vi "Kinimatics_Matrix_CoerceSize.vi"(9 "Columns":i32, 10 "Rows":i32, 11 "input matrix":T1) -> (0 "Coerced":bool, 3 "output matrix":T1)   [LabVIEW 2020, in "Swerve_Odometry_SEN.lvlib"]
doc: "Ensure a matrix is the size that is needed.\n\nInputs:\n - Input Matrix -- The matrix to be checked and resized if needed\n - Rows -- The expected number of rows\n - Columns -- The expected number of columns\n\nOutputs:\n - Output Matrix -- The potentially resized matrix\n - Coerced -- If TRUE, the matrix size was modified."
uses:
  <vilib>/Analysis/Matrix/Datatypes/RealMatrix.ctl
  Swerve_Odometry_SEN.lvlib
  <vilib>/Analysis/Matrix/NI_Matrix.lvlib
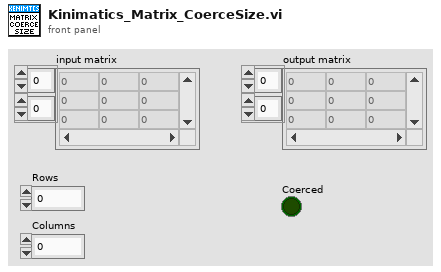
[diagram p1: front panel]
types:
  T1 = typedef "NI_Matrix.lvlib/RealMatrix.ctl" = dbl[][]
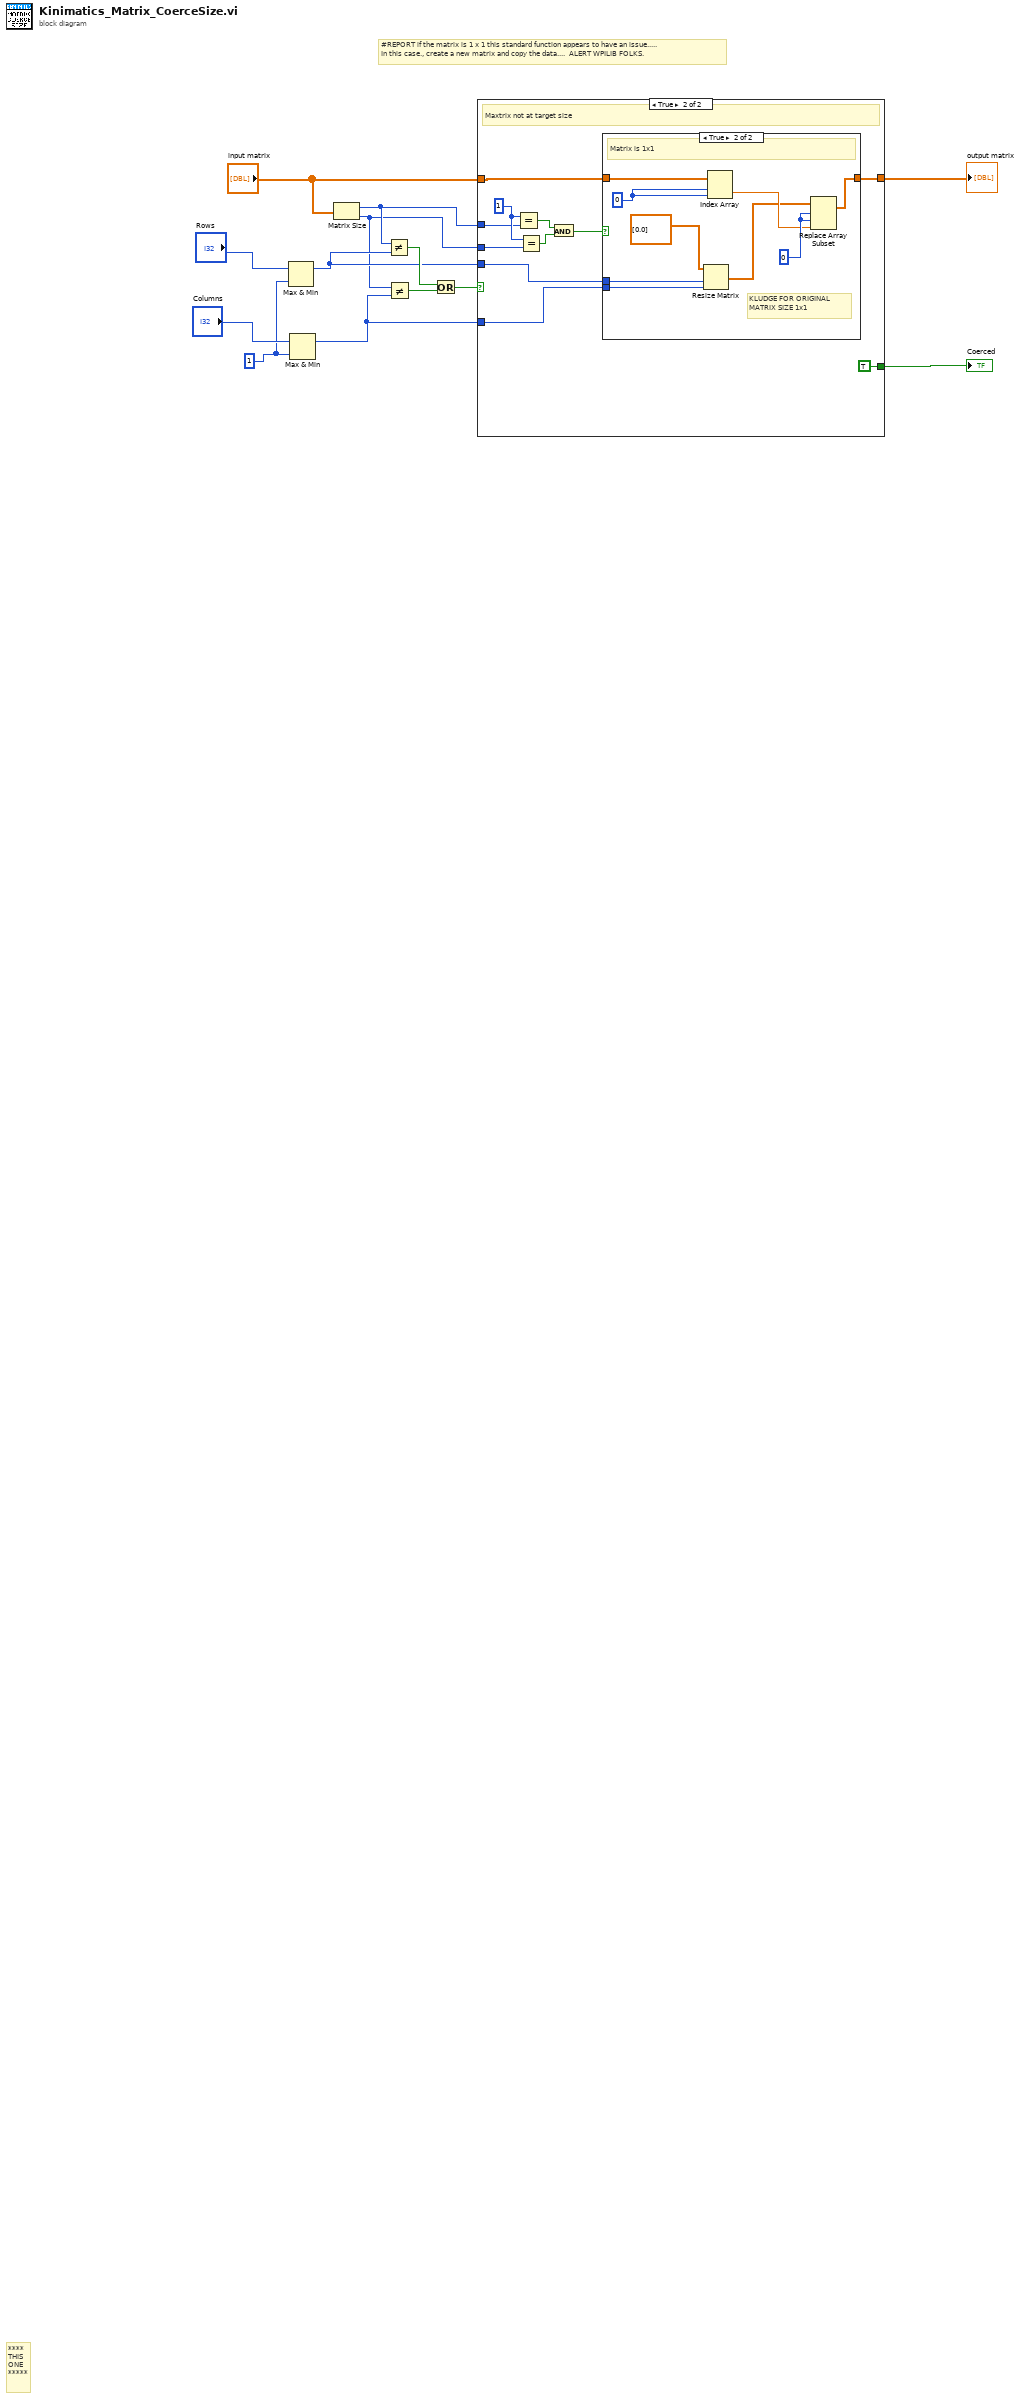
[diagram p0: block diagram]
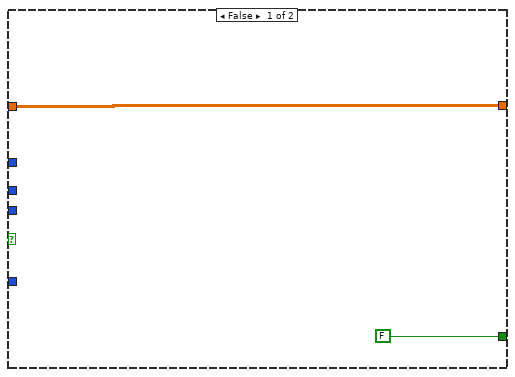
[diagram p2: hidden frame]
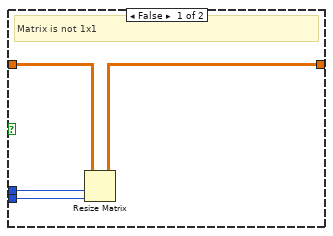
[diagram p3: hidden frame]
diagram:
  w6 = 1 ("y")
  # "#REPORT if the matrix is 1 x 1 this standard function appears to have an issue.....\nIn this case., create a new matrix and copy the data....  ALERT WPILIB FOLKS."
  # "****\nTHIS\nONE\n*****"
  n1 = Max & Min(x="Rows", y=w6) -> (max(x,y)=w5:i32)  [unwired: 1 out]
  n2 = Max & Min(x="Columns", y=w6) -> (max(x,y)=w4:i32)  [unwired: 1 out]
  n3 = Matrix Size(0:"input matrix") -> (1:w3:i32, 2:w2:i32)
  n4 = Not Equal?(x=w3, y=w5) -> (x != y?=w12:bool)
  n5 = Not Equal?(x=w2, y=w4) -> (x != y?=w11:bool)
  n6 = Or(x=w12, y=w11) -> (x .or. y?=w13:bool)
  n7 = case shown="True" w13 {
    tunnel: "input matrix" -> [w15 w18]
    tunnel: [w15 w17] -> w9
    tunnel: w5 -> [_ w20]
    tunnel: w4 -> [_ w19]
    tunnel: w3 -> [_ w25]
    tunnel: w2 -> [_ w24]
    tunnel: [FALSE TRUE] -> w1
    frame False {
    }
    frame True {
      w26 = 1 ("y")
      # "Maxtrix not at target size"
      n8 = Equal?(x=w26, y=w25) -> (x = y?=w22:bool)
      n9 = Equal?(x=w26, y=w24) -> (x = y?=w23:bool)
      n10 = And(x=w22, y=w23) -> (x .and. y?=w21:bool)
      n11 = case shown="True" w21 {
        tunnel: w20 -> [w28 w33]
        tunnel: w19 -> [w27 w32]
        tunnel: w18 -> [w29 w39]
        tunnel: [w30 w37] -> w17
        frame False {
          # "Matrix is not 1x1"
          n12 = Resize Matrix(1:w27, 2:w28, 4:w29) -> (0:w30:T1)
        }
        frame True {
          w36 = 0 ("disabled index (row)")
          w38 = 0 ("index (row)")
          # "KLUDGE FOR ORIGINAL\nMATRIX SIZE 1x1"
          # "Matrix is 1x1"
          n13 = Resize Matrix(1:w32, 2:w33, 4:T1 [[0.0]] ("matrix")) -> (0:w31:T1)
          n14 = Index Array(array=w39, index (row)=w38, index (col)=w38) -> (element=w35:dbl)
          n15 = Replace Array Subset(array=w31, new element=w35, index (row)=w36, index (col)=w36) -> (w37:T1)
        }
      }
    }
  }
  "output matrix" <- w9
  "Coerced" <- w1
